vi "Legend2009.vi"   [LabVIEW 2013]
uses:
  <vilib>/Heliosphere Research LLC/Advanced Plotting Toolkit/Advanced Plotting Toolkit.lvlib
types:
  T1 = typedef "Advanced Plotting Toolkit.lvlib/PlotID.ctl" = i32
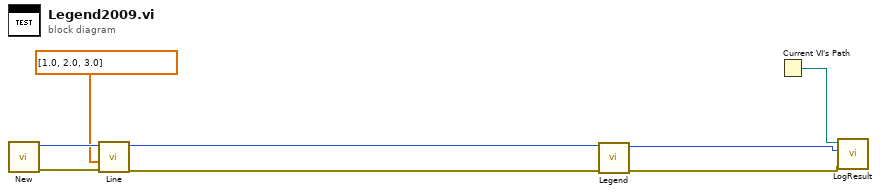
[diagram p0: block diagram]
diagram:
  n1 = call <vilib>:"New.vi"() -> ("error out"=w6:errorcluster, "Plot ID"=w7:T1)  [unwired: 10 in]
  n2 = call <vilib>:"Line.vi"("error in (no error)"=w6, "Y Data"=dbl[] [1.0, 2.0, 3.0], "Plot ID"=w7) -> ("error out"=w1:errorcluster, "Plot ID out"=w2:T1)  [unwired: 7 in]
  n3 = call <vilib>:"Legend.vi"("error in (no error)"=w1, "Plot ID"=w2) -> ("error out"=w4:errorcluster, "Plot ID Out"=w5:T1)  [unwired: 8 in]
  n4 = Current VI's Path() -> (path=w8:path)
  n5 = call "LogResult.vi"("Test Result"=w4, "Test Artifact"=w5, "VI Path"=w8) -> ()  [unwired: 9 in]
